vi "Update position.vi"(4 "Last position":cluster{"M1 pos":dbl, "M2 pos ":dbl}, 5 "Acquiring?":bool, 6 "Position 0":cluster{"M1 pos":dbl, "M2 pos ":dbl}, 7 "Motor":enum16{"All", "M1", "M2"}(ring), 8 "error in (no error)":errorcluster, 9 "Steps taken":i32, 10 "Direction M2":T1, 11 "Direction M1":T1) -> (0 "error out":errorcluster, 1 "Position out":cluster{"M1 pos":dbl, "M2 pos ":dbl})   [LabVIEW 2020]
uses:
  controls/Motor direction ---typedef.ctl
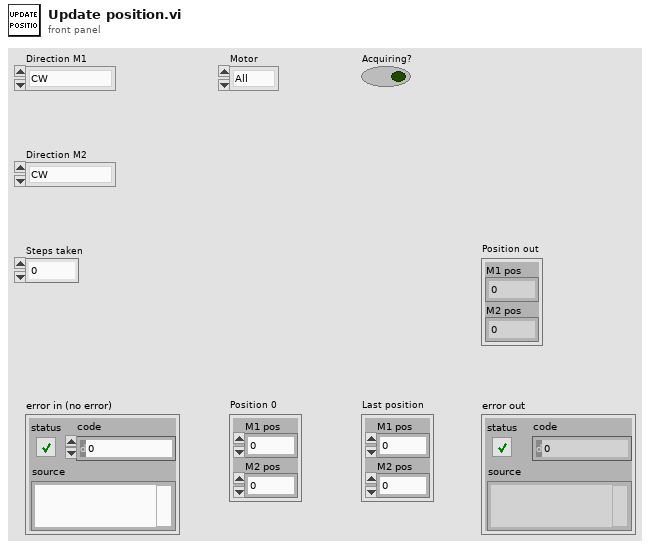
[diagram p1: front panel]
types:
  T1 = typedef "Motor direction ---typedef.ctl" = enum16{"CW", "CCW", "IDLE"}
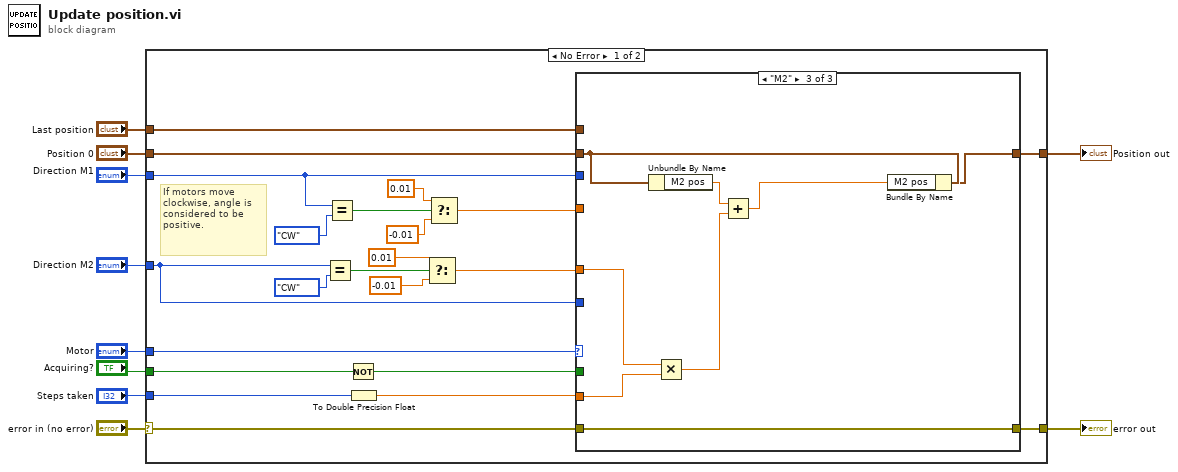
[diagram p0: block diagram]
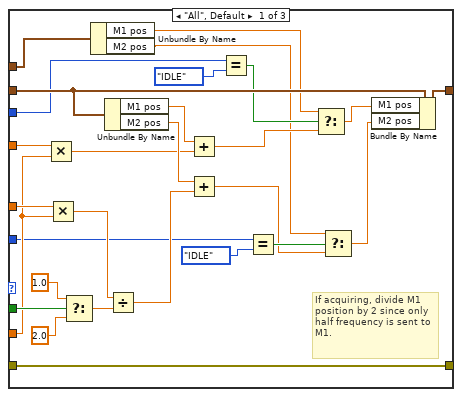
[diagram p2: hidden frame]
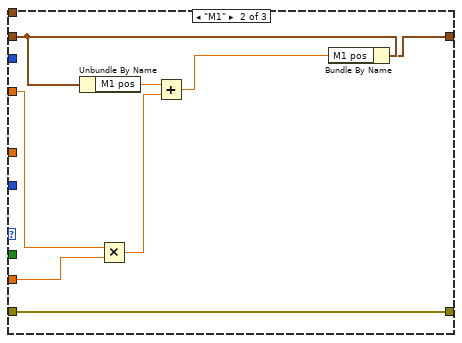
[diagram p3: hidden frame]
diagram:
  n1 = case shown="No Error" "error in (no error)" {
    selector: "error in (no error)" -> [w31 w78]
    tunnel: [w32 w78] -> w10
    tunnel: "Position 0" -> [w30 w77]
    tunnel: [w29 w77] -> w7
    tunnel: "Steps taken" -> [w28 _]
    tunnel: "Direction M1" -> [w14 _]
    tunnel: "Motor" -> [w22 _]
    tunnel: "Acquiring?" -> [w21 _]
    tunnel: "Direction M2" -> [w11 _]
    tunnel: "Last position" -> [w13 _]
    frame No Error {
      # "If motors move clockwise, angle is considered to be positive."
      n2 = Equal?(x=w11, y=Motor_direction_---typedef."CW") -> (x = y?=w20:bool)
      n3 = Equal?(x=w14, y=Motor_direction_---typedef."CW") -> (x = y?=w23:bool)
      n4 = Not(x=w21) -> (.not. x?=w16:bool)
      n5 = To Double Precision Float(number=w28) -> (double precision float=w27:dbl)
      n6 = Select(t=0.01 ("x"), s=w20, f=-0.01 ("x")) -> (s? t:f=w12:dbl)
      n7 = Select(t=0.01 ("x"), s=w23, f=-0.01 ("x")) -> (s? t:f=w15:dbl)
      n8 = case shown="\"M2\"" w22 {
        tunnel: w27 -> [w47 w67 w75]
        tunnel: w31 -> [w60 w68 w76]
        tunnel: [w60 w68 w76] -> w32
        tunnel: w15 -> [w59 w66 _]
        tunnel: w30 -> [w55 w63 w72]
        tunnel: [w54 w62 w70] -> w29
        tunnel: w16 -> [w51 _ _]
        tunnel: w12 -> [w48 _ w69]
        tunnel: w14 -> [w44 _ _]
        tunnel: w13 -> [w42 _ _]
        tunnel: w11 -> [w37 _ _]
        frame "All", Default {
          # "If acquiring, divide M1 position by 2 since only half frequency is sent to M1."
          n9 = Multiply(x=w59, y=w47) -> (x*y=w49:dbl)
          n10 = Multiply(x=w48, y=w47) -> (x*y=w46:dbl)
          n11 = Select(t=1.0, s=w51, f=2.0 ("y")) -> (s? t:f=w52:dbl)
          n12 = Unbundle By Name(w42) -> ("M1 pos"=w41:dbl, "M2 pos"=w35:dbl)
          n13 = Unbundle By Name(w55) -> ("M1 pos"=w58:dbl, "M2 pos"=w57:dbl)
          n14 = Divide(x=w46, y=w52) -> (x/y=w56:dbl)
          n15 = Add(x=w58, y=w49) -> (x+y=w40:dbl)
          n16 = Add(x=w57, y=w56) -> (x+y=w34:dbl)
          n17 = Equal?(x=w44, y=Motor_direction_---typedef."IDLE") -> (x = y?=w43:bool)
          n18 = Equal?(x=w37, y=Motor_direction_---typedef."IDLE") -> (x = y?=w36:bool)
          n19 = Select(t=w41, s=w43, f=w40) -> (s? t:f=w39:dbl)
          n20 = Select(t=w35, s=w36, f=w34) -> (s? t:f=w33:dbl)
          n21 = Bundle By Name(cluster=w55, "M1 pos"=w39, "M2 pos"=w33) -> (w54:cluster{"M1 pos":dbl, "M2 pos ":dbl})
        }
        frame "M1" {
          n22 = Unbundle By Name(w63) -> ("M1 pos"=w65:dbl)
          n23 = Multiply(x=w66, y=w67) -> (x*y=w64:dbl)
          n24 = Add(x=w65, y=w64) -> (x+y=w61:dbl)
          n25 = Bundle By Name(cluster=w63, "M1 pos"=w61) -> (w62:cluster{"M1 pos":dbl, "M2 pos ":dbl})
        }
        frame "M2" {
          n26 = Unbundle By Name(w72) -> ("M2 pos"=w74:dbl)
          n27 = Multiply(x=w69, y=w75) -> (x*y=w73:dbl)
          n28 = Add(x=w74, y=w73) -> (x+y=w71:dbl)
          n29 = Bundle By Name(cluster=w72, "M2 pos"=w71) -> (w70:cluster{"M1 pos":dbl, "M2 pos ":dbl})
        }
      }
    }
    frame Error {
    }
  }
  "error out" <- w10
  "Position out" <- w7
